vi "laser tuning derivative control.vi"(8 "lower limit":dbl=3.7, 9 "upper limit":dbl=3.7) -> (1 "c8 voltage":dbl, 2 "laser task out":refnum<k21>, 3 "germanium task out":refnum<k21>)   [LabVIEW 2018]
uses:
  <vilib>/DAQmx/write.llb/DAQmx Write (Analog DBL 1Chan 1Samp).vi
  0a1fad13-b885-4eab-b2d2-ceeba4e32cbd.vi
  <vilib>/DAQmx/read.llb/DAQmx Read (Analog DBL 1Chan 1Samp).vi
  <vilib>/Analysis/baseanly.llb/Mean (DBL).vi
  <vilib>/DAQmx/create/channels.llb/DAQmx Create Channel (AO-Voltage-Basic).vi
  <vilib>/DAQmx/miscellaneous.llb/DAQmx Fill In Error Info.vi
  <vilib>/DAQmx/create/channels.llb/DAQmx Create Channel (AI-Voltage-Basic).vi
  <vilib>/ptbypt/NI_PtbyPt.lvlib
  <vilib>/Analysis/NI_AALBase.lvlib
panel:
  out "Derivative":dbl(graph)
  out "Average":dbl(graph)
  out "current voltage":dbl
  out "diode voltage":dbl
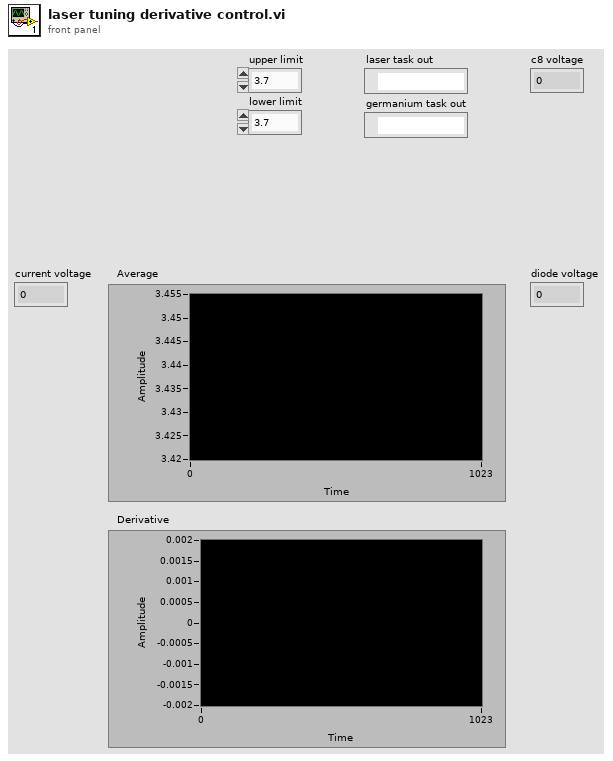
[diagram p1: front panel]
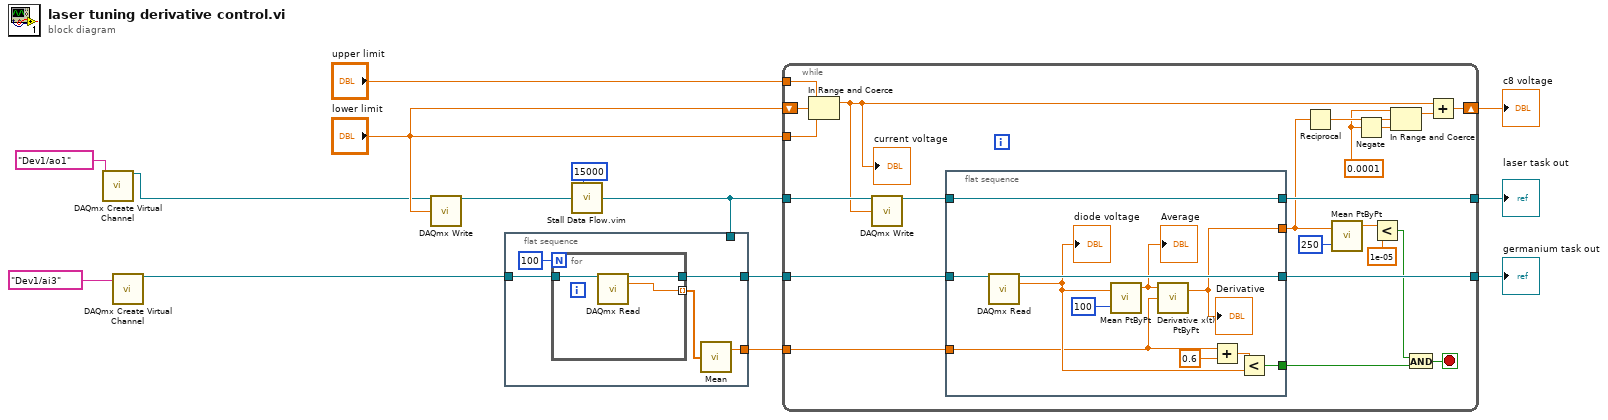
[diagram p0: block diagram]
diagram:
  n1 = call-poly <vilib>:"DAQmx Create Virtual Channel.vi"("physical channels"=tag "Dev1/ao1") -> ("task out"=w2:refnum<k21>)  [unwired: 13 in, 1 out]
  n2 = call-poly <vilib>:"DAQmx Create Virtual Channel.vi"("physical channels"=tag "Dev1/ai3") -> ("task out"=w1:refnum<k21>)  [unwired: 13 in, 1 out]
  n3 = call-poly <vilib>:"DAQmx Write.vi"("task/channels in"=w2, "data"="lower limit") -> ("task out"=w14:refnum<k21>)  [unwired: 11 in, 2 out]
  n4 = flat-sequence {
    tunnel: w1 -> [w19]
    tunnel: [w18] -> w7
    tunnel: [w15] -> w5
    tunnel: w6 -> [_]
    frame #0 {
      n5 = for {
        N: 100 -> [_]
        tunnel: [w20] -> w16 mode=indexing
        tunnel: w19 -> [w22]
        tunnel: [w21] -> w18
        n6 = call-poly <vilib>:"DAQmx Read.vi"("task/channels in"=w22) -> ("task out"=w21:refnum<k21>, "data"=w20:dbl)  [unwired: 12 in, 1 out]
      }
      n7 = call-poly <vilib>:"Mean.vi"("X"=w16) -> ("mean"=w15:dbl)  [unwired: 1 out]
    }
  }
  n8 = call "Stall Data Flow.vim"("value in"=w14, "milliseconds to wait"=u32 15000) -> ("value out"=w6:refnum<k21>)  [unwired: 1 out]
  n9 = while {
    shift-right: [w41] -> w10
    shift-left: "lower limit" -> [w40]
    tunnel: "upper limit" -> [w34]
    tunnel: "lower limit" -> [w33]
    tunnel: w7 -> [w42]
    tunnel: [w43] -> w11
    tunnel: w5 -> [w30]
    tunnel: w6 -> [w44]
    tunnel: [w31] -> w12
    stop <- w27 stop-if-true
    w36 = 0.0001 ("limit")
    n10 = In Range and Coerce(upper limit=w34, x=w40, lower limit=w33) -> (coerced(x)=w39:dbl)  [unwired: 1 out]
    "current voltage" <- w39
    n11 = call-poly <vilib>:"DAQmx Write.vi"("task/channels in"=w44, "data"=w39) -> ("task out"=w32:refnum<k21>)  [unwired: 11 in, 2 out]
    n12 = flat-sequence {
      tunnel: [w55] -> w43
      tunnel: w42 -> [w54]
      tunnel: w32 -> [w52]
      tunnel: [w52] -> w31
      tunnel: w30 -> [w46]
      tunnel: [w48] -> w23
      tunnel: [w47] -> w28
      frame #0 {
        n13 = call-poly <vilib>:"DAQmx Read.vi"("task/channels in"=w54) -> ("task out"=w55:refnum<k21>, "data"=w50:dbl)  [unwired: 12 in, 1 out]
        "diode voltage" <- w50
        n14 = call <vilib>:"Mean PtByPt.vi"("x"=w50, "sample length"=100) -> ("mean"=w51:dbl)  [unwired: 2 in, 1 out]
        "Average" <- w51
        n15 = call <vilib>:"Derivative x(t) PtByPt.vi"("initial condition"=w46, "x"=w51) -> ("dx/dt"=w47:dbl)  [unwired: 2 in, 1 out]
        "Derivative" <- w47
        n16 = Add(x=w46, y=0.6) -> (x+y=w49:dbl)
        n17 = Less?(x=w49, y=w50) -> (x < y?=w48:bool)
      }
    }
    n18 = Reciprocal(x=w28) -> (1/x=w38:dbl)
    n19 = call <vilib>:"Mean PtByPt.vi"("x"=w28, "sample length"=250) -> ("mean"=w25:dbl)  [unwired: 2 in, 1 out]
    n20 = Negate(x=w36) -> (-x=w35:dbl)
    n21 = Less?(x=w25, y=1e-05 ("x")) -> (x < y?=w24:bool)
    n22 = In Range and Coerce(upper limit=w36, x=w38, lower limit=w35) -> (coerced(x)=w37:dbl)  [unwired: 1 out]
    n23 = And(x=w24, y=w23) -> (x .and. y?=w27:bool)
    n24 = Add(x=w39, y=w37) -> (x+y=w41:dbl)
  }
  "laser task out" <- w12
  "germanium task out" <- w11
  "c8 voltage" <- w10
